vi "Count repeated primes.vi"(8 "Max total":i32[](array[numeric]), 9 "Previous total":i32[](array[numeric]), 10 "Numbers to look for":i64[](array[numeric])=[2, 3, 5, 7, 11], 11 "Array":i64[](array[numeric])) -> (0 "Below max reps":bool, 1 "Total found":i32[](array[numeric]), 3 "Found times":i32[](array[numeric]))   [LabVIEW 2015]
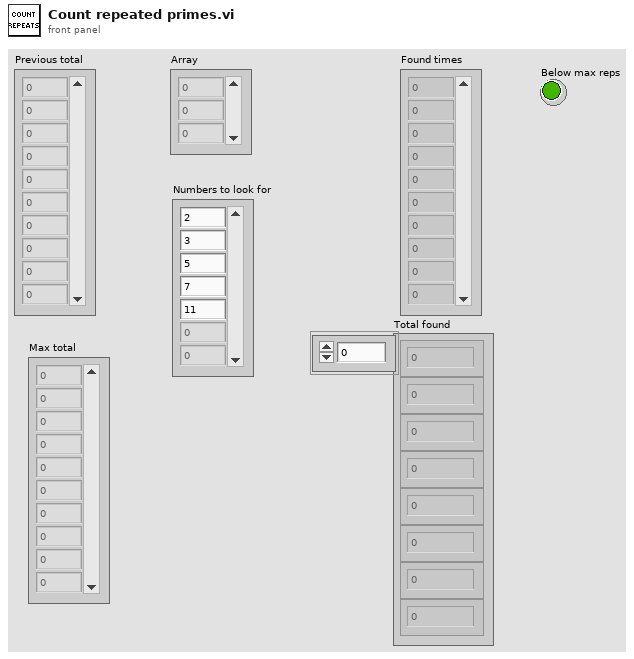
[diagram p1: front panel]
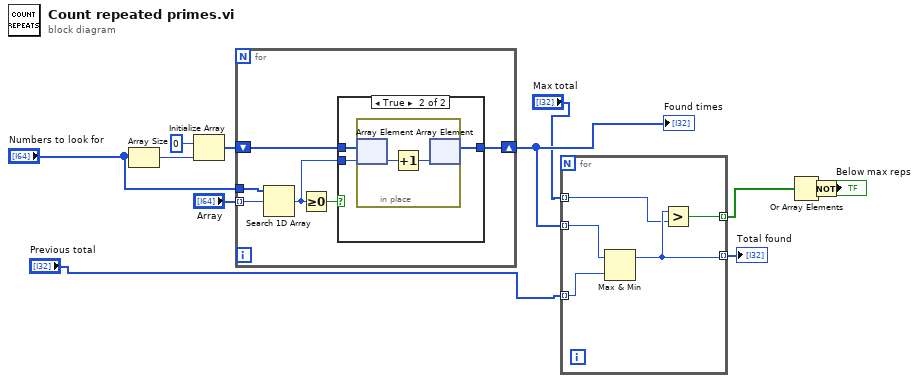
[diagram p0: block diagram]
diagram:
  n1 = Array Size(array="Numbers to look for") -> (size(s)=w12:i32)
  n2 = Initialize Array(0, w12) -> (w10:i32[])
  n3 = for {
    shift-right: [w14] -> w7
    shift-left: w10 -> [w16]
    tunnel: "Array" -> [w18] mode=indexing
    tunnel: "Numbers to look for" -> [w13]
    n4 = Search 1D Array(1D array=w13, element=w18) -> (index of element=w15:i32)  [unwired: 1 in]
    n5 = Greater Or Equal To 0?(x=w15) -> (x >= 0?=w17:bool)
    n6 = case shown="True" w17 {
      tunnel: w16 -> [w19 w22]
      tunnel: w15 -> [_ w21]
      tunnel: [w19 w20] -> w14
      frame False {
      }
      frame True {
        n7 = in-place {
          n8 = in-place-array #1(w22, w21) -> (w24:i32)
          n9 = Increment(x=w24) -> (x+1=w23:i32)
          n10 = in-place-array #1(w23) -> (w20:i32[])  [unwired: 1 out]
        }
      }
    }
  }
  "Found times" <- w7
  n11 = for {
    tunnel: w7 -> [w29] mode=indexing
    tunnel: "Previous total" -> [w28] mode=indexing
    tunnel: [w27] -> w5 mode=indexing
    tunnel: "Max total" -> [w26] mode=indexing
    tunnel: [w25] -> w3 mode=indexing
    n12 = Max & Min(x=w29, y=w28) -> (max(x,y)=w27:i32)  [unwired: 1 out]
    n13 = Greater?(x=w27, y=w26) -> (0:w25:bool)
  }
  "Total found" <- w5
  n14 = Or Array Elements(Boolean array=w3) -> (logical OR=w2:bool)
  n15 = Not(x=w2) -> (.not. x?=→"Below max reps":bool)
